vi "MainLauncher.vi"() -> ()   [LabVIEW 2024, in "Launcher_DTU.lvlib"]
uses:
  Launcher_DTU.lvlib
  Controls_Main/Main_typedef_DTU.ctl
  SubVI/Global 1.vi
  Modules/Settings/Setting_Screen.lvlib
  Modules/LaunchTest/LaunchTest.lvlib
  Modules/MANUAL_MODE/MANUAL_MODE.lvlib
panel:
  in  "Manual mode":bool
  in  "RunScreen":bool
  in  "Exit":bool
  in  "Settings":bool
  out "error constant 2":errorcluster
  in  "error constant":errorcluster
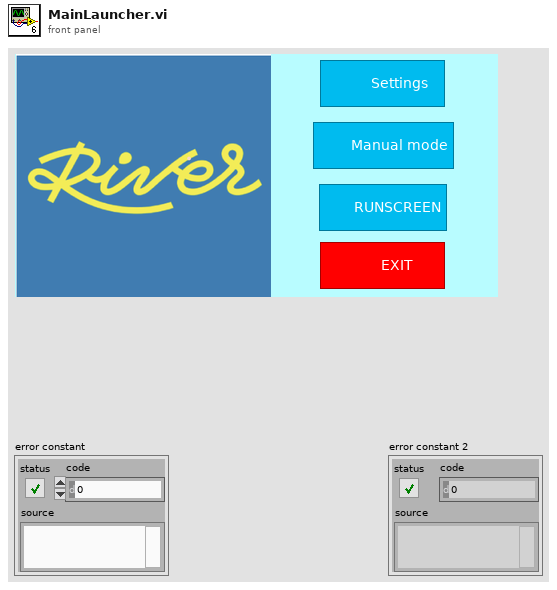
[diagram p1: front panel]
types:
  T1 = typedef "Launcher_DTU.lvlib/Main_typedef_DTU.ctl" = enum16{"Init", "Poll", "Login", "Settings", "Manual", "RunScreen", "Exit"}
  T2 = cluster{"Log member":enum16{"Admin", "Operator"}, "Operator name":string}
  T3 = enum32{"Invalid", "Standard", "Closed", "Hidden", "Minimized", "Maximized"}
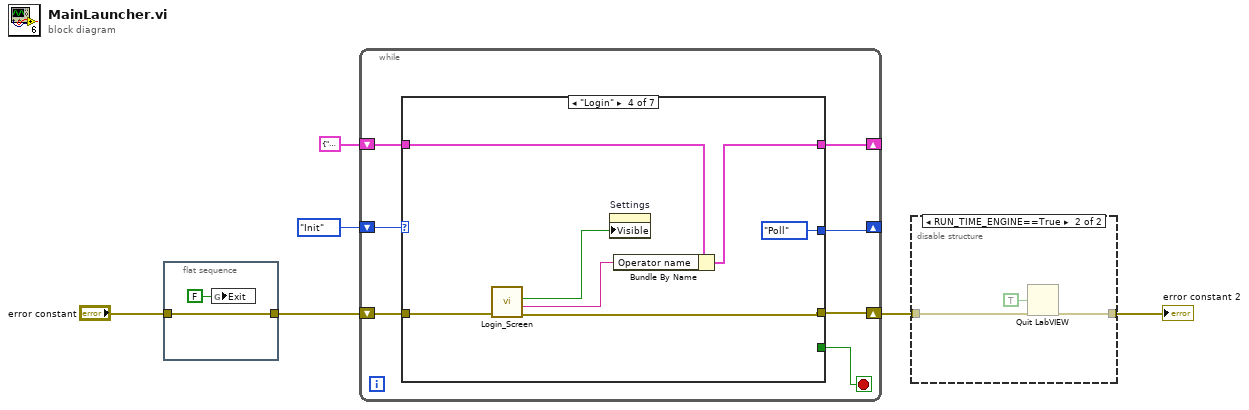
[diagram p0: block diagram]
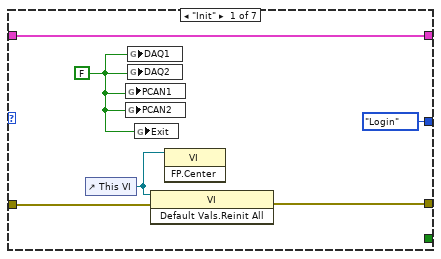
[diagram p3: hidden frame]
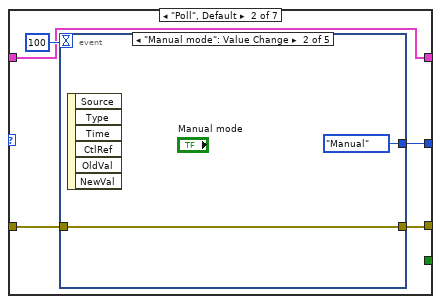
[diagram p4: hidden frame]
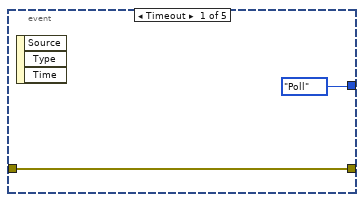
[diagram p5: hidden frame]
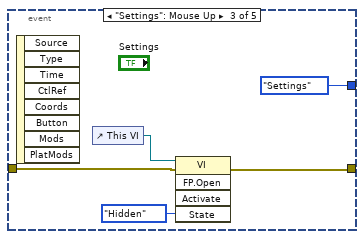
[diagram p6: hidden frame]
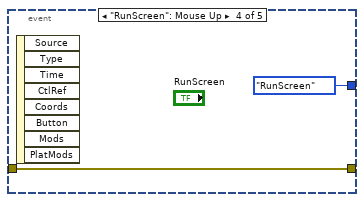
[diagram p7: hidden frame]
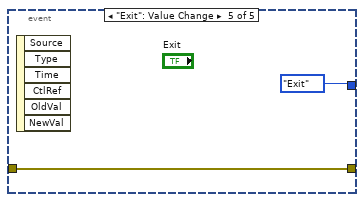
[diagram p8: hidden frame]
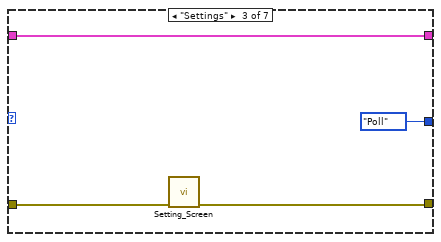
[diagram p9: hidden frame]
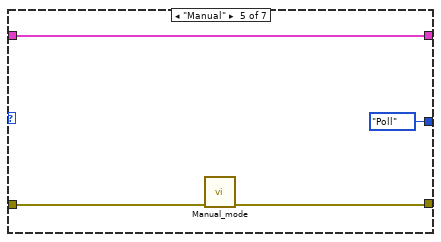
[diagram p10: hidden frame]
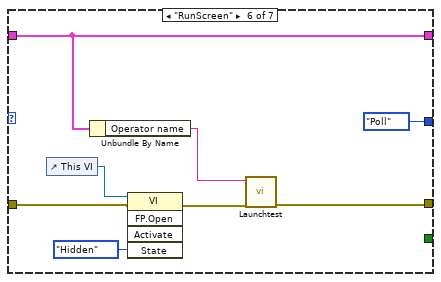
[diagram p11: hidden frame]
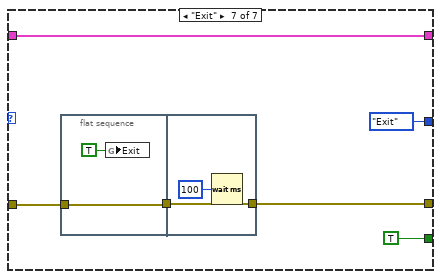
[diagram p12: hidden frame]
diagram:
  n1 = flat-sequence {
    tunnel: [w8] -> w2
    tunnel: "error constant" -> [w8]
    frame #0 {
      n2 = global write "Global 1.vi" "Exit"(FALSE ("Exit")) -> ()
    }
  }
  n3 = while {
    shift-right: [w14] -> w5
    shift-left: w2 -> [w15]
    shift-right: [w11] -> _
    shift-left: Main_typedef_DTU."Init" ("Enum_Main") -> [w12]
    shift-right: [w9] -> _
    shift-left: T2 {"Log member"=enum."Admin", "Operator name"=""} -> [w10]
    stop <- w13 stop-if-true
    n4 = case shown="\"Login\"" w12 {
      tunnel: w15 -> [w21 w26 w43 w49 w54 w59 w66]
      tunnel: [w20 w25 w42 w48 w52 w62 w65] -> w14
      tunnel: [_ _ _ _ _ _ TRUE] -> w13
      tunnel: [Main_typedef_DTU."Login" ("Enum_Main") w23 Main_typedef_DTU."Poll" ("Enum_Main") Main_typedef_DTU."Poll" ("Enum_Main") Main_typedef_DTU."Poll" ("Enum_Main") Main_typedef_DTU."Poll" ("Enum_Main") Main_typedef_DTU."Exit" ("Enum_Main")] -> w11
      tunnel: w10 -> [w18 w22 w41 w50 w53 w57 w67]
      tunnel: [w18 w22 w41 w47 w53 w57 w67] -> w9
      frame "Init" {
        w17 = FALSE
        n5 = control-ref of="This VI"() -> (w19:refnum<vi>)
        n6 = global write "Global 1.vi" "PCAN1"(w17) -> ()
        n7 = global write "Global 1.vi" "PCAN2"(w17) -> ()
        n8 = global write "Global 1.vi" "DAQ1"(w17) -> ()
        n9 = global write "Global 1.vi" "DAQ2"(w17) -> ()
        n10 = global write "Global 1.vi" "Exit"(w17) -> ()
        n11 = invoke class="VI" method="Default Vals.Reinit All"(reference=w19, error in=w21) -> (error out=w20:errorcluster)  [unwired: 1 in, 2 out]
        n12 = invoke class="VI" method="FP.Center"(reference=w19) -> ()  [unwired: 2 in, 3 out]
      }
      frame "Poll", Default {
        n13 = event shown="[1] \"Manual mode\": Value Change" {
          selector: _ -> [_ _ _ _ _]
          dyn-events: _ -> [_ _ _ _ _]
          timeout: 100 -> [_ _ _ _ _]
          tunnel: [w28 w29 w34 w37 w39] -> w25
          tunnel: w26 -> [w28 w29 w35 w37 w39]
          tunnel: [Main_typedef_DTU."Poll" ("Enum_Main") Main_typedef_DTU."Manual" ("Enum_Main") Main_typedef_DTU."Settings" ("Enum_Main") Main_typedef_DTU."RunScreen" ("Enum_Main") Main_typedef_DTU."Exit" ("Enum_Main")] -> w23
          event Timeout {
            n14 = event-data() -> ()  [unwired: 1 in, 3 out]
          }
          event "Manual mode": Value Change {
            n15 = event-data() -> ()  [unwired: 1 in, 6 out]
          }
          event "Settings": Mouse Up {
            n16 = event-data() -> ()  [unwired: 1 in, 8 out]
            n17 = control-ref of="This VI"() -> (w33:refnum<vi>)
            n18 = invoke class="VI" method="FP.Open"(reference=w33, error in=w35, "State"=T3."Hidden") -> (error out=w34:errorcluster)  [unwired: 2 in, 4 out]
          }
          event "RunScreen": Mouse Up {
            n19 = event-data() -> ()  [unwired: 1 in, 8 out]
          }
          event "Exit": Value Change {
            n20 = event-data() -> ()  [unwired: 1 in, 6 out]
          }
        }
      }
      frame "Settings" {
        n21 = call "Setting_Screen.vi"("error in (no error)"=w43) -> ("error in (out)"=w42:errorcluster)  [unwired: 10 in]
      }
      frame "Login" {
        n22 = call "Login_Screen.vi"("error constant"=w49) -> ("error constant 2"=w48:errorcluster, "Operator Name 2"=w46:string, "Admin?"=w45:bool)  [unwired: 8 in]
        n23 = property on="Settings" class="Bool"("Visible"=w45) -> ()  [unwired: 2 in, 2 out]
        n24 = Bundle By Name(cluster=w50, "Operator name"=w46) -> (w47:T2)
      }
      frame "Manual" {
        n25 = call "Manual_mode.vi"("error in (no error)"=w54) -> ("error in (out)"=w52:errorcluster)  [unwired: 10 in]
      }
      frame "RunScreen" {
        n26 = control-ref of="This VI"() -> (w61:refnum<vi>)
        n27 = Unbundle By Name(w57) -> ("Operator name"=w56:string)
        n28 = invoke class="VI" method="FP.Open"(reference=w61, error in=w59, "State"=T3."Hidden") -> (error out=w58:errorcluster)  [unwired: 2 in, 4 out]
        n29 = call "Launchtest.vi"("error in (no error)"=w58, "Operator name"=w56) -> ("error in (out)"=w62:errorcluster)  [unwired: 9 in]
      }
      frame "Exit" {
        n30 = flat-sequence {
          tunnel: w66 -> [w70]
          tunnel: [w70] -> w64
          tunnel: [w72] -> w65
          tunnel: w64 -> [w72]
          frame #0 {
            n31 = global write "Global 1.vi" "Exit"(TRUE ("Exit")) -> ()
          }
          frame #1 {
            n32 = Wait (ms)(milliseconds to wait=u32 100) -> ()  [unwired: 1 out]
          }
        }
      }
    }
  }
  n33 = disable-structure shown="RUN_TIME_ENGINE==True" {
    disable-tunnel: w5 -> [w73 w75]
    disable-tunnel: [w73 w75] -> w4
    frame condition #0 (active) {
    }
    frame condition #1 {
      n34 = Quit LabVIEW(quit? (T)=TRUE) -> ()
    }
  }
  "error constant 2" <- w4
